vi "Write Headers to CSV File.vi"(6 "Array":string[](array[string])=["Time", "Throttle % ", "Speed Summary", "Torque Summary", "Power", "Gear Ratio", "Engine Speed", "Engine Torque", "L Speed", "R Speed", "H Speed", "L Torque ", "R Torque ", "H Torque ", "Intercooler_In_T", "Intercooler_Out_T", "Exhaust_T", "Oil_T", "Coolant_Inlet_T", "Coolant_Outlet_T", "Basement_T", "T Spare 1", "T Spare 2", "T Spare 3", "T Spare 4", "T Spare 5", "T Spare 6", "T Spare 7", "T Spare 8", "Coolant-In_P", "Coolant-Out_P", "Exhaust_P", "Oil_P", "Intercooler-In_P", "Intercooler-Out_P", "Misc_P ", "P Spare 1", "P Spare 2", "P Spare 3", "P Spare 4", "Engine RPM "], 8 "error in (no error)":errorcluster, 10 "Headers":string[](array[string]), 11 "file path":path) -> (0 "error out":errorcluster, 3 "LogFile Refnum":refnum<file>)   [LabVIEW 2018]
doc: "This VI closes file reference"
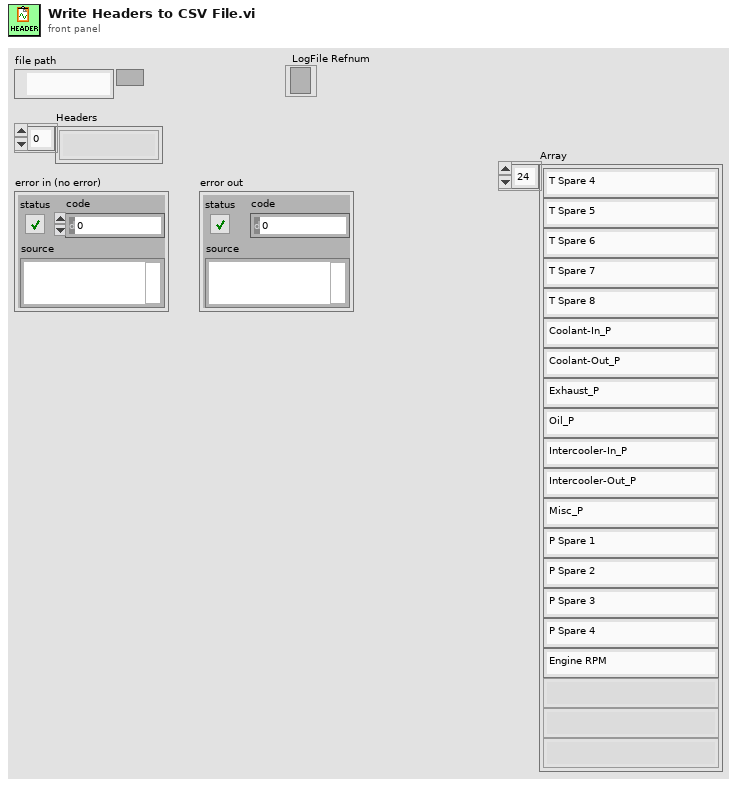
[diagram p1: front panel]
types:
  T1 = enum16{"open", "replace", "create", "open or create", "replace or create", "replace or create with confirmation"}
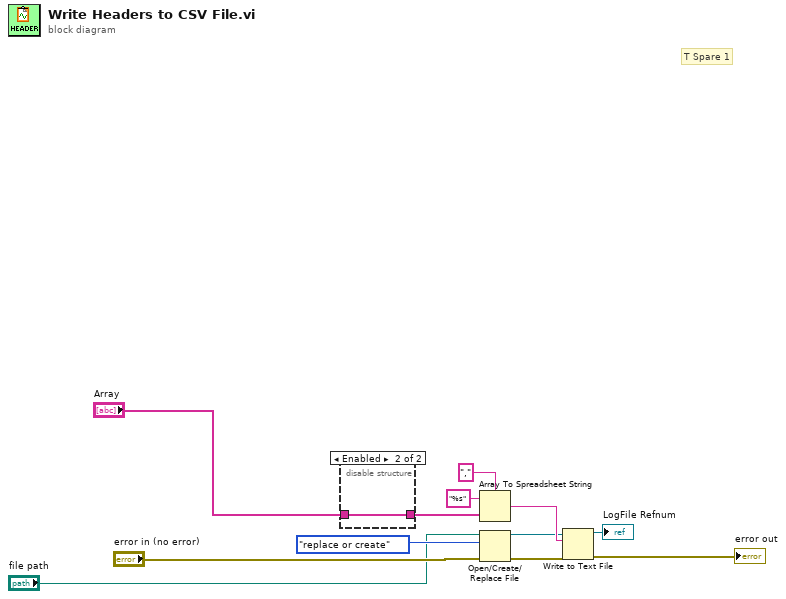
[diagram p0: block diagram]
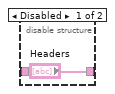
[diagram p2: hidden frame]
diagram:
  # "T Spare 1"
  n1 = disable-structure shown="Enabled" {
    disable-tunnel: ["Headers" w14] -> w7
    disable-tunnel: "Array" -> [_ w14]
    frame Disabled {
    }
    frame Enabled {
    }
  }
  n2 = Array To Spreadsheet String(delimiter (Tab)=",", array=w7, 3:"%s" ("format string")) -> (spreadsheet string=w8:string)
  n3 = Open/Create/Replace File(file path (use dialog)="file path", error in="error in (no error)", operation (0:open)=T1."replace or create") -> (refnum out=w6:refnum<file>, error out=w3:errorcluster)  [unwired: 3 in, 1 out]
  n4 = Write to Text File(file (use dialog)=w6, text=w8, error in=w3) -> (refnum out=→"LogFile Refnum":refnum<file>, error out=→"error out":errorcluster)  [unwired: 1 in, 1 out]
